vi "Do.vi"(8 "error in":errorcluster, 10 "Actor in":refnum<class "Actor.lvclass">, 11 "Generate Event Msg":refnum<class "Generate Event Msg.lvclass">) -> (0 "error out":errorcluster, 2 "Actor out":refnum<class "Actor.lvclass">)   [LabVIEW 2020, in "Event Source.lvlib" / "Generate Event Msg.lvclass"]
doc: "This VI delivers the message to the actor by calling the appropriate method(s) on the actor."
uses:
  Generate Event Msg.lvclass
  <vilib>/ActorFramework/Actor/Actor.lvclass
  Generate Event Msg.lvclass/Generate Event Msg.ctl
  Event Source/Event Source.lvclass
  9ef47adc-f318-494c-9b8b-6df3216d6863.vi
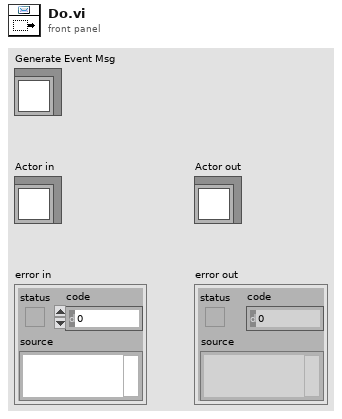
[diagram p1: front panel]
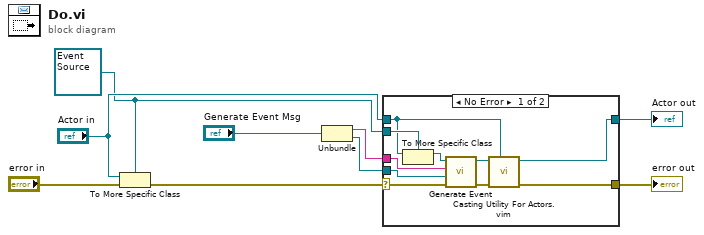
[diagram p0: block diagram]
diagram:
  w3 = refnum<class "Event Source.lvclass"> refnum ("Actor in")
  n1 = To More Specific Class(target class=w3, reference="Actor in", error in="error in") -> (error out=w7:errorcluster)  [unwired: 1 out]
  n2 = Unbundle("Generate Event Msg") -> (w2:string, w1:refnum<class "Event Data.lvclass">)
  n3 = case shown="No Error" w7 {
    selector: w7 -> [w19 w21]
    tunnel: [w13 w21] -> w6
    tunnel: [w14 w20] -> w5
    tunnel: "Actor in" -> [w16 w20]
    tunnel: w3 -> [w17 _]
    tunnel: w2 -> [w11 _]
    tunnel: w1 -> [w10 _]
    frame No Error {
      n4 = To More Specific Class(target class=w17, reference=w16) -> (specific class reference=w18:refnum<class "Event Source.lvclass">)  [unwired: 1 in, 1 out]
      n5 = call-dynamic "Generate Event.vi"("Error In"=w19, "Event Data"=w10, "Event Name"=w11, "Event Source In"=w18) -> ("Error Out"=w12:errorcluster, "Event Source Out"=w15:refnum<class "Event Source.lvclass">)  [unwired: 6 in]
      n6 = call "Casting Utility For Actors.vim"("type"=w16, "error in (no error)"=w12, "Actor in"=w15) -> ("error out"=w13:errorcluster, "Actor out"=w14:refnum<class "Actor.lvclass">)  [unwired: 7 in]
    }
    frame Error {
      # "If type check fails, pass the original object out again."
    }
  }
  "error out" <- w6
  "Actor out" <- w5
